vi "Read Specified Address Dispense Parameters.vi"(0 "VISA resource name":refnum<visa-resource-name>, 5 "Memory Location (ccc)":i32 min=0 max=399 step=1 format="%03.0f", 11 "error in (no error)":errorcluster) -> (4 "VISA resource name out":refnum<visa-resource-name>, 6 "Pressure":dbl, 8 "Dispense Time":dbl, 10 "Vacuum":dbl, 15 "error out":errorcluster)   [LabVIEW 2018, in "EFD Ultimus V.lvlib"]
doc: "Reads the dispense pressure, time and vacuum of the specified address. This command will update the LCD screen to the specified memory location. 'D0' is the number zero (0). CONFIGURED TO WORK WITH PRESSURE SET TO PSI, VAC SET TO inH2O. If different units are used, VI has to be adjusted for different limits. \n\nHost Format: E8ccc\nccc: The 3 digit memory location from 0-399. The dispenser will automatically limit value to prevent any errors.\n\nReturn Format: D0PDppppDTtttttVCvvvv\npppp: The four digit pressure setting excluding the decimal point. This is a unit less value. The valid pressure ranges and decimal point are determined by the pressure units currently selected in the dispenser. \nttttt: The five digit dispense time value excluding the decimal point. The valid range is 0.0000 to 9.9999 seconds. \npppp: The four digit vacuum setting excluding the decimal point. This is a unit less value. The valid vacuum ranges and decimal point are determined by the vacuum units currently selected in the dispenser."
uses:
  EFD Ultimus V.lvlib
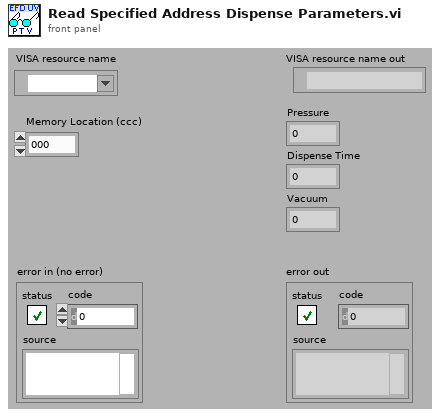
[diagram p1: front panel]
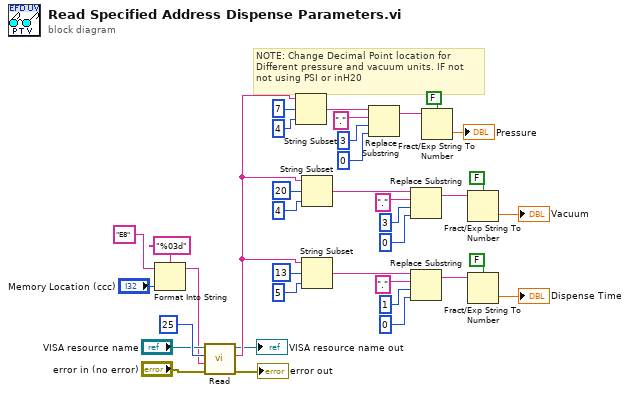
[diagram p0: block diagram]
diagram:
  # "NOTE: Change Decimal Point location for \nDifferent pressure and vacuum units. IF not\nnot using PSI or inH20"
  n1 = Format Into String(format string="%03d", initial string="E8" ("string"), "Memory Location (ccc)") -> (resulting string=w6:string)  [unwired: 1 in, 1 out]
  n2 = call "Read.vi"("error in (no error)"="error in (no error)", "Command To Write"=w6, "Bytes to Read (11)"=u32 25 ("Bytes to Read from Buffer"), "VISA resource name"="VISA resource name") -> ("error out"=→"error out":errorcluster, "Ultimus V Feedback Data"=w24:string, "VISA resource name out"=→"VISA resource name out":refnum<visa-resource-name>)  [unwired: 5 out]
  n3 = String Subset(string=w24, offset (0)=7, length (rest)=4 ("length (rest)")) -> (substring=w26:string)
  n4 = String Subset(string=w24, offset (0)=20, length (rest)=4 ("length (rest)")) -> (substring=w37:string)
  n5 = String Subset(string=w24, offset (0)=13, length (rest)=5 ("length (rest)")) -> (substring=w10:string)
  n6 = Replace Substring(2:0 ("length (len. of substring)"), 3:3 ("offset (0)"), 4:"." ("substring (\"\")"), 5:w26) -> (1:w30:string)  [unwired: 1 out]
  n7 = Replace Substring(2:0 ("length (len. of substring)"), 3:3 ("offset (0)"), 4:"." ("substring (\"\")"), 5:w37) -> (1:w33:string)  [unwired: 1 out]
  n8 = Replace Substring(2:0 ("length (len. of substring)"), 3:1 ("offset (0)"), 4:"." ("substring (\"\")"), 5:w10) -> (1:w14:string)  [unwired: 1 out]
  n9 = Fract/Exp String To Number(use system decimal point (T)=FALSE, string=w30) -> (number=→"Pressure":dbl)  [unwired: 3 out]
  n10 = Fract/Exp String To Number(use system decimal point (T)=FALSE, string=w33) -> (number=→"Vacuum":dbl)  [unwired: 3 out]
  n11 = Fract/Exp String To Number(use system decimal point (T)=FALSE, string=w14) -> (number=→"Dispense Time":dbl)  [unwired: 3 out]
